vi "cm_Close Time Display VIs.vi"(8 "error in (no error)":errorcluster, 11 "Time Display Ref in":refnum<vi>[](array[refnum])) -> (0 "error out":errorcluster, 3 "Time Display Ref out":refnum<vi>[](array[refnum]))   [LabVIEW 2012, in "Channel Monitor.xctl"]
uses:
  Channel Monitor.xctl
  <userlib>/AMC/Queue Registry/TypeDefs/amc_QueueRegistryMethod.ctl
  <userlib>/AMC/Queue Registry/TypeDefs/amc_QueueRegistryProperties.ctl
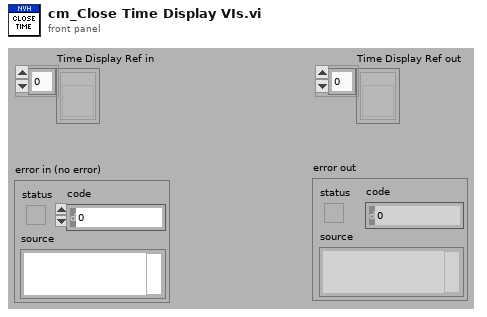
[diagram p1: front panel]
types:
  T1 = typedef "amc_QueueRegistryProperties.ctl" = cluster{"Name":string}
  T2 = typedef "amc_QueueRegistryMethod.ctl" = enum16{"Initialize", "Add Queue", "Set Properties", "Get Queue by Index", "Get Queue by Name", "Remove Queue", "Remove All Queues"}
  T3 = typedef "amc_Message Queue.ctl" = refnum<queue>
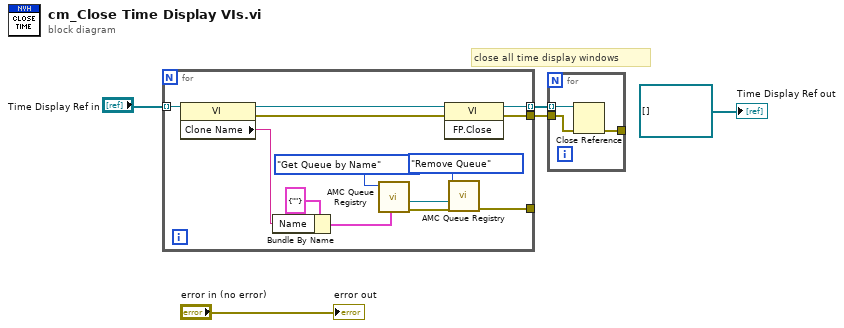
[diagram p0: block diagram]
diagram:
  # "close all time display windows"
  n1 = for {
    tunnel: "Time Display Ref in" -> [w17] mode=indexing
    tunnel: [w18] -> w4 mode=indexing
    tunnel: [w8] -> _
    tunnel: [w7] -> w1
    n2 = property class="VI"(reference=w17) -> (reference out=w16:refnum<vi>, error out=w6:errorcluster, "Clone Name"=w11:string)  [unwired: 1 in]
    n3 = Bundle By Name(cluster=T1 {"Name"=""} ("Properties in"), "Name"=w11) -> (w10:T1)
    n4 = call <userlib>:"AMC Queue Registry.vi"("Properties in"=w10, "Method"=amc_QueueRegistryMethod."Get Queue by Name") -> ("error out"=w9:errorcluster, "Message Queue out"=w13:T3)  [unwired: 4 in, 4 out]
    n5 = invoke class="VI" method="FP.Close"(reference=w16, error in=w6) -> (reference out=w18:refnum<vi>, error out=w7:errorcluster)  [unwired: 1 in, 1 out]
    n6 = call <userlib>:"AMC Queue Registry.vi"("error in (no error)"=w9, "Message Queue in"=w13, "Method"=amc_QueueRegistryMethod."Remove Queue") -> ("error out"=w8:errorcluster)  [unwired: 3 in, 5 out]
  }
  n7 = for {
    tunnel: w4 -> [w21] mode=indexing
    tunnel: w1 -> [w20]
    tunnel: [w19] -> _
    n8 = Close Reference(reference=w21, error in (no error)=w20) -> (error out=w19:errorcluster)
  }
  "Time Display Ref out" <- refnum<vi>[] [] ("Time Display Ref")
  "error out" <- "error in (no error)"
